vi "RelayBoard_16in16out_ZQ.vi"() -> ()   [LabVIEW 2013]
uses:
  <vilib>/Instr/_visa.llb/VISA Configure Serial Port (Instr).vi
panel:
  out "数组 2":bool[](array[boolean])
  out "数组":bool[](array[boolean])
  out "连接状态":bool
  in  "全部断开":bool
  in  "全部闭合":bool
  in  "OUT 16":bool
  in  "OUT 15":bool
  in  "OUT 14":bool
  in  "OUT 13":bool
  in  "OUT 12":bool
  in  "OUT 11":bool
  in  "OUT 10":bool
  in  "OUT 9":bool
  in  "OUT 8":bool
  in  "OUT 7":bool
  in  "OUT 6":bool
  in  "OUT 5":bool
  in  "OUT 4":bool
  in  "OUT 3":bool
  in  "打开端口":bool
  in  "停止":bool
  in  "OUT 2":bool
  in  "OUT 1":bool
  in  "VISA resource name":refnum<visa-resource-name> caption="VISA资源名称"
  # "X1"
  # "X2"
  # "X3"
  # "X4"
  # "X5"
  # "X6"
  # "X7"
  # "X8"
  # "X9"
  # "X10"
  # "X11"
  # "X12"
  # "X13"
  # "X14"
  # "X15"
  # "X16"
  # "X1"
  # "X2"
  # "X3"
  # "X4"
  # "X5"
  # "X6"
  # "X7"
  # "X8"
  # "X9"
  # "X10"
  # "X11"
  # "X12"
  # "X13"
  # "X14"
  # "X15"
  # "X16"
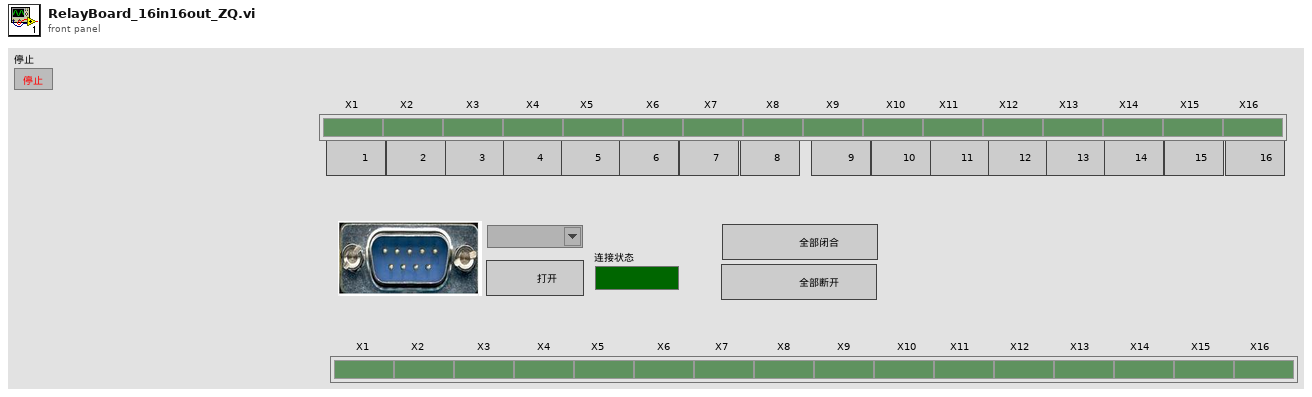
[diagram p1: front panel]
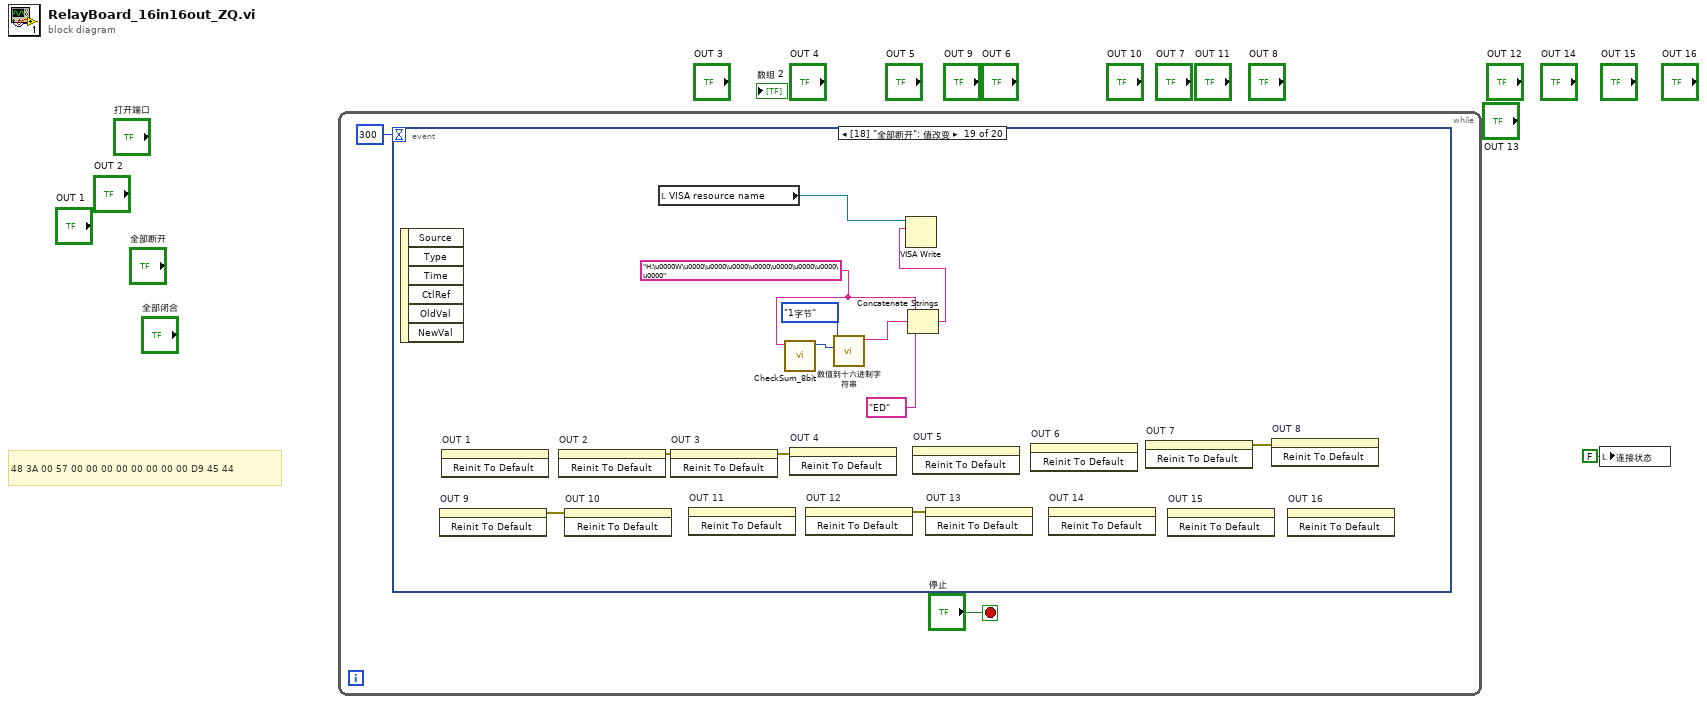
[diagram p0: block diagram]
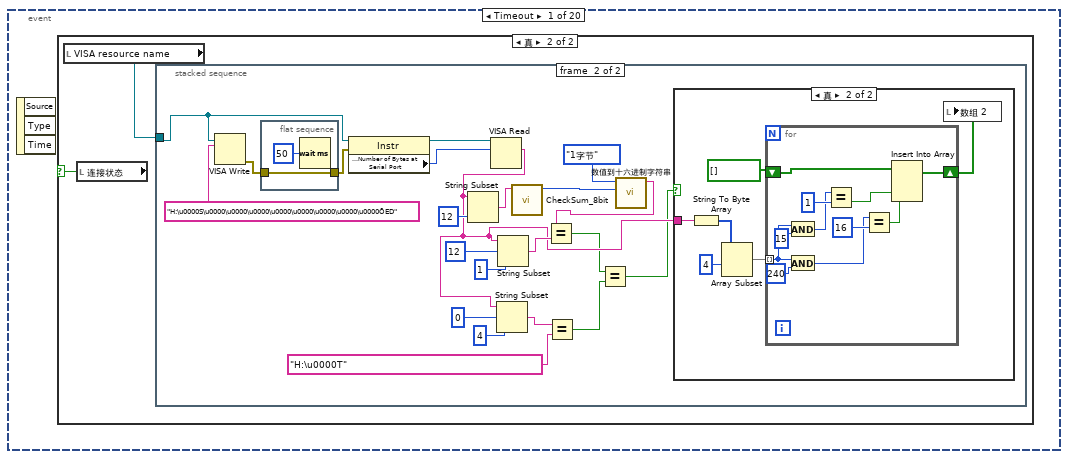
[diagram p2: hidden frame]
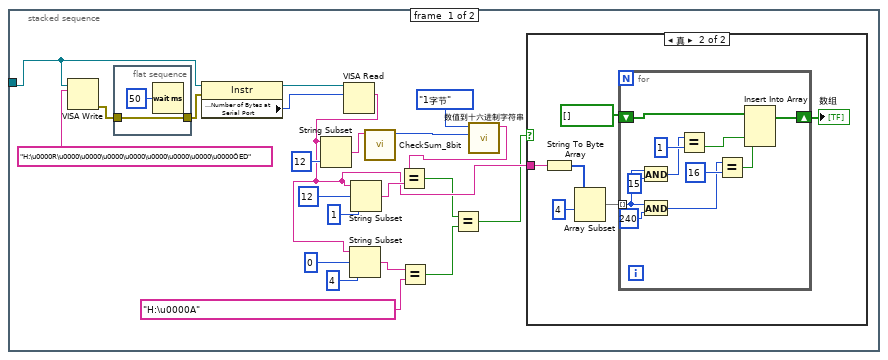
[diagram p4: hidden frame]
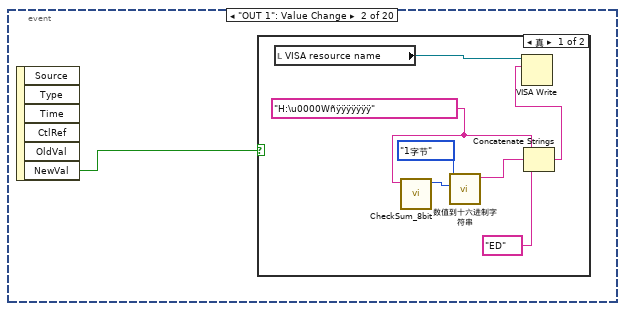
[diagram p7: hidden frame]
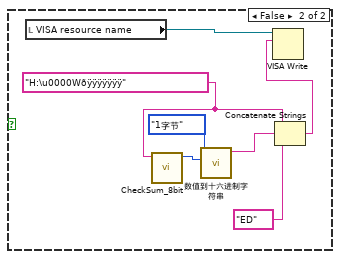
[diagram p8: hidden frame]
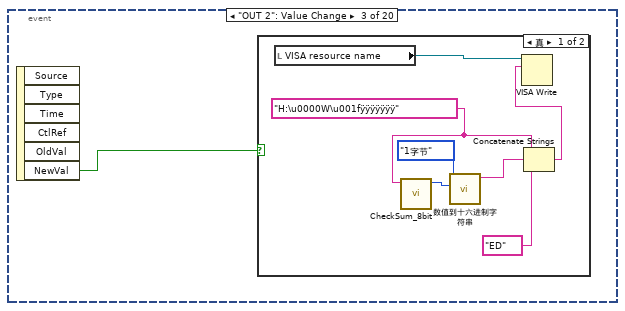
[diagram p9: hidden frame]
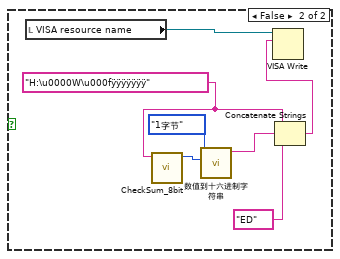
[diagram p10: hidden frame]
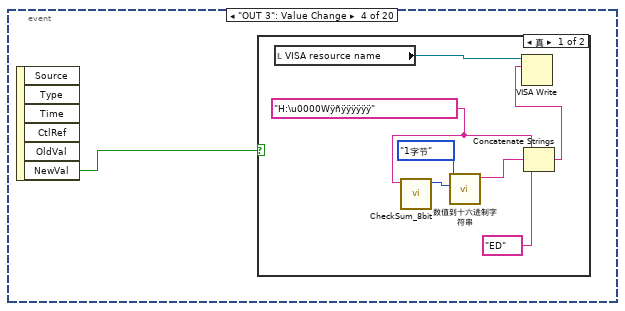
[diagram p11: hidden frame]
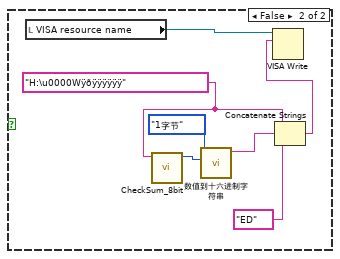
[diagram p12: hidden frame]
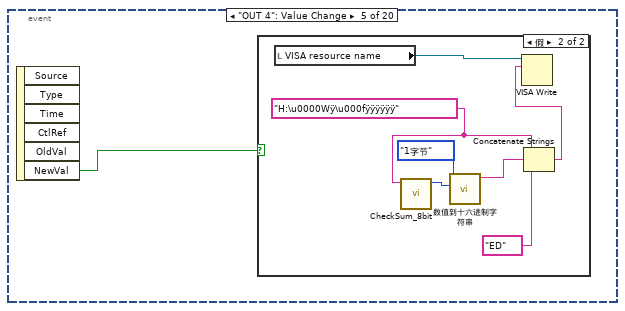
[diagram p13: hidden frame]
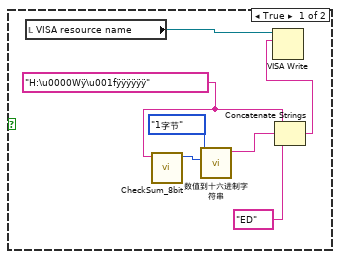
[diagram p14: hidden frame]
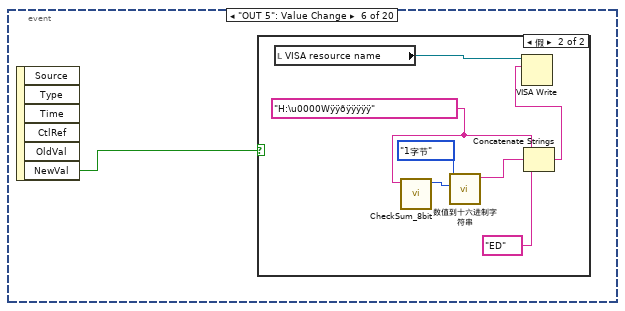
[diagram p15: hidden frame]
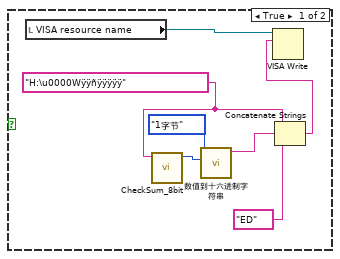
[diagram p16: hidden frame]
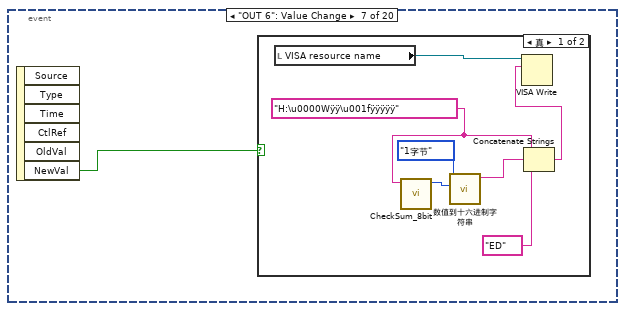
[diagram p17: hidden frame]
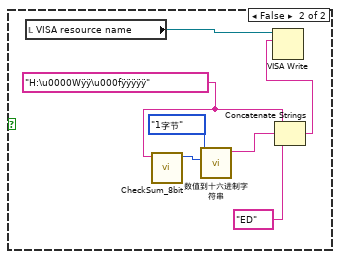
[diagram p18: hidden frame]
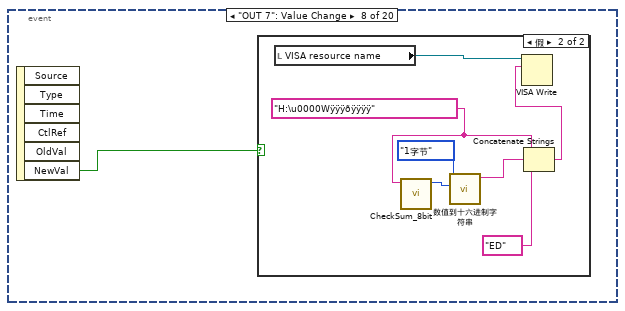
[diagram p19: hidden frame]
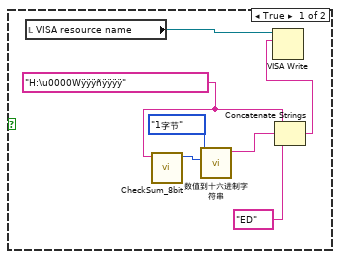
[diagram p20: hidden frame]
diagram:
  # "48 3A 00 57 00 00 00 00 00 00 00 00 D9 45 44"
  n1 = while {
    stop <- "停止" stop-if-true
    n2 = event shown="[18] \"全部断开\": 值改变" {
      selector: _ -> [_ _ _ _ _ _ _ _ _ _ _ _ _ _ _ _ _ _ _ _]
      dyn-events: _ -> [_ _ _ _ _ _ _ _ _ _ _ _ _ _ _ _ _ _ _ _]
      timeout: 300 -> [_ _ _ _ _ _ _ _ _ _ _ _ _ _ _ _ _ _ _ _]
      event Timeout {
        n3 = event-data() -> ()  [unwired: 1 in, 3 out]
        n4 = local read "连接状态"() -> (w4:bool)
        n5 = case shown="真" w4 {
          frame False {
          }
          frame True {
            n6 = local read "VISA resource name"() -> (w5:refnum<visa-resource-name>)
            n7 = stacked-sequence {
              tunnel: w5 -> [w22 w63]
              frame #0 {
                n8 = VISA Write(VISA resource name=w22, write buffer="H:\u0000R\u0000\u0000\u0000\u0000\u0000\u0000\u0000\u0000ÔED" ("写入缓冲区")) -> (error out=w23:errorcluster)  [unwired: 1 in, 2 out]
                n9 = flat-sequence {
                  tunnel: [w28] -> w24
                  tunnel: w23 -> [w28]
                  frame #0 {
                    n10 = Wait (ms)(milliseconds to wait=u32 50 ("等待时间（毫秒）")) -> ()  [unwired: 1 out]
                  }
                }
                n11 = property class="Instr"(reference=w22, error in=w24) -> (reference out=w27:refnum<visa-resource-name>, "Serial Settings:Number of Bytes at Serial Port"=w26:u32)  [unwired: 1 out]
                n12 = VISA Read(VISA resource name=w27, byte count=w26) -> (read buffer=w11:string)  [unwired: 1 in, 3 out]
                n13 = String Subset(string=w11, length (rest)=12 ("长度（剩余）")) -> (substring=w17:string)  [unwired: 1 in]
                n14 = String Subset(string=w11, offset (0)=0 ("偏移量(0)"), length (rest)=4 ("长度（剩余）")) -> (substring=w10:string)
                n15 = String Subset(string=w11, offset (0)=12 ("偏移量(0)"), length (rest)=1 ("长度（剩余）")) -> (substring=w18:string)
                n16 = call "CheckSum_8bit.vi"("字符串"=w17) -> ("和"=w15:u32)  [unwired: 10 in]
                n17 = Equal?(x=w10, y="H:\u0000A" ("写入缓冲区")) -> (x = y?=w7:bool)
                n18 = call "数值到十六进制字符串.vi"("Numeric"=w15, "转换字节数"=enum16{"1字节", "2字节", "4字节", "3字节"}."1字节") -> ("转换结果"=w14:string)  [unwired: 8 in, 1 out]
                n19 = Equal?(x=w14, y=w18) -> (x = y?=w8:bool)
                n20 = Equal?(x=w8, y=w7) -> (x = y?=w6:bool)
                n21 = case shown="真" w6 {
                  tunnel: w11 -> [_ w35]
                  frame False {
                  }
                  frame True {
                    n22 = String To Byte Array(string=w35) -> (unsigned byte array=w34:u8[])
                    n23 = Array Subset(array=w34, index=4 ("索引")) -> (w32:u8[])  [unwired: 1 in]
                    n24 = for {
                      tunnel: w32 -> [w39] mode=indexing
                      shift-right: [w41] -> w30
                      shift-left: bool[] [] -> [w44]
                      n25 = And(x=w39, y=u8 15) -> (x .and. y?=w37:u8)
                      n26 = And(x=w39, y=u8 240) -> (x .and. y?=w36:u8)
                      n27 = Equal?(x=w37, y=u8 1) -> (x = y?=w43:bool)
                      n28 = Equal?(x=w36, y=u8 16) -> (x = y?=w42:bool)
                      n29 = Insert Into Array(array=w44, new element #1=w43, new element #2=w42) -> (w41:bool[])  [unwired: 1 in]
                    }
                    "数组" <- w30
                  }
                }
              }
              frame #1 {
                n30 = VISA Write(VISA resource name=w63, write buffer="H:\u0000S\u0000\u0000\u0000\u0000\u0000\u0000\u0000\u0000ÕED" ("写入缓冲区")) -> (error out=w64:errorcluster)  [unwired: 1 in, 2 out]
                n31 = flat-sequence {
                  tunnel: [w69] -> w65
                  tunnel: w64 -> [w69]
                  frame #0 {
                    n32 = Wait (ms)(milliseconds to wait=u32 50 ("等待时间（毫秒）")) -> ()  [unwired: 1 out]
                  }
                }
                n33 = property class="Instr"(reference=w63, error in=w65) -> (reference out=w68:refnum<visa-resource-name>, "Serial Settings:Number of Bytes at Serial Port"=w67:u32)  [unwired: 1 out]
                n34 = VISA Read(VISA resource name=w68, byte count=w67) -> (read buffer=w52:string)  [unwired: 1 in, 3 out]
                n35 = String Subset(string=w52, length (rest)=12 ("长度（剩余）")) -> (substring=w58:string)  [unwired: 1 in]
                n36 = String Subset(string=w52, offset (0)=0 ("偏移量(0)"), length (rest)=4 ("长度（剩余）")) -> (substring=w51:string)
                n37 = String Subset(string=w52, offset (0)=12 ("偏移量(0)"), length (rest)=1 ("长度（剩余）")) -> (substring=w59:string)
                n38 = call "CheckSum_8bit.vi"("字符串"=w58) -> ("和"=w56:u32)  [unwired: 10 in]
                n39 = Equal?(x=w51, y="H:\u0000T" ("写入缓冲区")) -> (x = y?=w48:bool)
                n40 = call "数值到十六进制字符串.vi"("Numeric"=w56, "转换字节数"=enum16{"1字节", "2字节", "4字节", "3字节"}."1字节") -> ("转换结果"=w55:string)  [unwired: 8 in, 1 out]
                n41 = Equal?(x=w55, y=w59) -> (x = y?=w49:bool)
                n42 = Equal?(x=w49, y=w48) -> (x = y?=w47:bool)
                n43 = case shown="真" w47 {
                  tunnel: w52 -> [_ w76]
                  frame False {
                  }
                  frame True {
                    n44 = String To Byte Array(string=w76) -> (unsigned byte array=w75:u8[])
                    n45 = Array Subset(array=w75, index=4 ("索引")) -> (w73:u8[])  [unwired: 1 in]
                    n46 = for {
                      tunnel: w73 -> [w80] mode=indexing
                      shift-right: [w82] -> w71
                      shift-left: bool[] [] -> [w85]
                      n47 = And(x=w80, y=u8 15) -> (x .and. y?=w78:u8)
                      n48 = And(x=w80, y=u8 240) -> (x .and. y?=w77:u8)
                      n49 = Equal?(x=w78, y=u8 1) -> (x = y?=w84:bool)
                      n50 = Equal?(x=w77, y=u8 16) -> (x = y?=w83:bool)
                      n51 = Insert Into Array(array=w85, new element #1=w84, new element #2=w83) -> (w82:bool[])  [unwired: 1 in]
                    }
                    n52 = local write "数组 2"(w71) -> ()
                  }
                }
              }
            }
          }
        }
      }
      event "OUT 1": Value Change {
        n53 = event-data() -> ("NewVal"=w88:bool)  [unwired: 1 in, 5 out]
        n54 = case shown="真" w88 {
          frame True {
            w89 = "H:\u0000Wñÿÿÿÿÿÿÿ" ("写入缓冲区")
            n55 = local read "VISA resource name"() -> (w95:refnum<visa-resource-name>)
            n56 = call "CheckSum_8bit.vi"("字符串"=w89) -> ("和"=w94:u32)  [unwired: 10 in]
            n57 = call "数值到十六进制字符串.vi"("Numeric"=w94, "转换字节数"=enum16{"1字节", "2字节", "4字节", "3字节"}."1字节") -> ("转换结果"=w92:string)  [unwired: 8 in, 1 out]
            n58 = Concatenate Strings(w89, w92, "ED" ("写入缓冲区")) -> (w90:string)
            n59 = VISA Write(VISA resource name=w95, write buffer=w90) -> ()  [unwired: 1 in, 3 out]
          }
          frame False {
            w96 = "H:\u0000Wðÿÿÿÿÿÿÿ" ("写入缓冲区")
            n60 = local read "VISA resource name"() -> (w102:refnum<visa-resource-name>)
            n61 = call "CheckSum_8bit.vi"("字符串"=w96) -> ("和"=w101:u32)  [unwired: 10 in]
            n62 = call "数值到十六进制字符串.vi"("Numeric"=w101, "转换字节数"=enum16{"1字节", "2字节", "4字节", "3字节"}."1字节") -> ("转换结果"=w99:string)  [unwired: 8 in, 1 out]
            n63 = Concatenate Strings(w96, w99, "ED" ("写入缓冲区")) -> (w97:string)
            n64 = VISA Write(VISA resource name=w102, write buffer=w97) -> ()  [unwired: 1 in, 3 out]
          }
        }
      }
      event "OUT 2": Value Change {
        n65 = event-data() -> ("NewVal"=w103:bool)  [unwired: 1 in, 5 out]
        n66 = case shown="真" w103 {
          frame True {
            w104 = "H:\u0000W\u001fÿÿÿÿÿÿÿ" ("写入缓冲区")
            n67 = local read "VISA resource name"() -> (w110:refnum<visa-resource-name>)
            n68 = call "CheckSum_8bit.vi"("字符串"=w104) -> ("和"=w109:u32)  [unwired: 10 in]
            n69 = call "数值到十六进制字符串.vi"("Numeric"=w109, "转换字节数"=enum16{"1字节", "2字节", "4字节", "3字节"}."1字节") -> ("转换结果"=w107:string)  [unwired: 8 in, 1 out]
            n70 = Concatenate Strings(w104, w107, "ED" ("写入缓冲区")) -> (w105:string)
            n71 = VISA Write(VISA resource name=w110, write buffer=w105) -> ()  [unwired: 1 in, 3 out]
          }
          frame False {
            w111 = "H:\u0000W\u000fÿÿÿÿÿÿÿ" ("写入缓冲区")
            n72 = local read "VISA resource name"() -> (w117:refnum<visa-resource-name>)
            n73 = call "CheckSum_8bit.vi"("字符串"=w111) -> ("和"=w116:u32)  [unwired: 10 in]
            n74 = call "数值到十六进制字符串.vi"("Numeric"=w116, "转换字节数"=enum16{"1字节", "2字节", "4字节", "3字节"}."1字节") -> ("转换结果"=w114:string)  [unwired: 8 in, 1 out]
            n75 = Concatenate Strings(w111, w114, "ED" ("写入缓冲区")) -> (w112:string)
            n76 = VISA Write(VISA resource name=w117, write buffer=w112) -> ()  [unwired: 1 in, 3 out]
          }
        }
      }
      event "OUT 3": Value Change {
        n77 = event-data() -> ("NewVal"=w118:bool)  [unwired: 1 in, 5 out]
        n78 = case shown="真" w118 {
          frame True {
            w119 = "H:\u0000Wÿñÿÿÿÿÿÿ" ("写入缓冲区")
            n79 = local read "VISA resource name"() -> (w125:refnum<visa-resource-name>)
            n80 = call "CheckSum_8bit.vi"("字符串"=w119) -> ("和"=w124:u32)  [unwired: 10 in]
            n81 = call "数值到十六进制字符串.vi"("Numeric"=w124, "转换字节数"=enum16{"1字节", "2字节", "4字节", "3字节"}."1字节") -> ("转换结果"=w122:string)  [unwired: 8 in, 1 out]
            n82 = Concatenate Strings(w119, w122, "ED" ("写入缓冲区")) -> (w120:string)
            n83 = VISA Write(VISA resource name=w125, write buffer=w120) -> ()  [unwired: 1 in, 3 out]
          }
          frame False {
            w126 = "H:\u0000Wÿðÿÿÿÿÿÿ" ("写入缓冲区")
            n84 = local read "VISA resource name"() -> (w132:refnum<visa-resource-name>)
            n85 = call "CheckSum_8bit.vi"("字符串"=w126) -> ("和"=w131:u32)  [unwired: 10 in]
            n86 = call "数值到十六进制字符串.vi"("Numeric"=w131, "转换字节数"=enum16{"1字节", "2字节", "4字节", "3字节"}."1字节") -> ("转换结果"=w129:string)  [unwired: 8 in, 1 out]
            n87 = Concatenate Strings(w126, w129, "ED" ("写入缓冲区")) -> (w127:string)
            n88 = VISA Write(VISA resource name=w132, write buffer=w127) -> ()  [unwired: 1 in, 3 out]
          }
        }
      }
      event "OUT 4": Value Change {
        n89 = event-data() -> ("NewVal"=w133:bool)  [unwired: 1 in, 5 out]
        n90 = case shown="假" w133 {
          frame True {
            w134 = "H:\u0000Wÿ\u001fÿÿÿÿÿÿ" ("写入缓冲区")
            n91 = local read "VISA resource name"() -> (w140:refnum<visa-resource-name>)
            n92 = call "CheckSum_8bit.vi"("字符串"=w134) -> ("和"=w139:u32)  [unwired: 10 in]
            n93 = call "数值到十六进制字符串.vi"("Numeric"=w139, "转换字节数"=enum16{"1字节", "2字节", "4字节", "3字节"}."1字节") -> ("转换结果"=w137:string)  [unwired: 8 in, 1 out]
            n94 = Concatenate Strings(w134, w137, "ED" ("写入缓冲区")) -> (w135:string)
            n95 = VISA Write(VISA resource name=w140, write buffer=w135) -> ()  [unwired: 1 in, 3 out]
          }
          frame False {
            w141 = "H:\u0000Wÿ\u000fÿÿÿÿÿÿ" ("写入缓冲区")
            n96 = local read "VISA resource name"() -> (w147:refnum<visa-resource-name>)
            n97 = call "CheckSum_8bit.vi"("字符串"=w141) -> ("和"=w146:u32)  [unwired: 10 in]
            n98 = call "数值到十六进制字符串.vi"("Numeric"=w146, "转换字节数"=enum16{"1字节", "2字节", "4字节", "3字节"}."1字节") -> ("转换结果"=w144:string)  [unwired: 8 in, 1 out]
            n99 = Concatenate Strings(w141, w144, "ED" ("写入缓冲区")) -> (w142:string)
            n100 = VISA Write(VISA resource name=w147, write buffer=w142) -> ()  [unwired: 1 in, 3 out]
          }
        }
      }
      event "OUT 5": Value Change {
        n101 = event-data() -> ("NewVal"=w148:bool)  [unwired: 1 in, 5 out]
        n102 = case shown="假" w148 {
          frame True {
            w149 = "H:\u0000Wÿÿñÿÿÿÿÿ" ("写入缓冲区")
            n103 = local read "VISA resource name"() -> (w155:refnum<visa-resource-name>)
            n104 = call "CheckSum_8bit.vi"("字符串"=w149) -> ("和"=w154:u32)  [unwired: 10 in]
            n105 = call "数值到十六进制字符串.vi"("Numeric"=w154, "转换字节数"=enum16{"1字节", "2字节", "4字节", "3字节"}."1字节") -> ("转换结果"=w152:string)  [unwired: 8 in, 1 out]
            n106 = Concatenate Strings(w149, w152, "ED" ("写入缓冲区")) -> (w150:string)
            n107 = VISA Write(VISA resource name=w155, write buffer=w150) -> ()  [unwired: 1 in, 3 out]
          }
          frame False {
            w156 = "H:\u0000Wÿÿðÿÿÿÿÿ" ("写入缓冲区")
            n108 = local read "VISA resource name"() -> (w162:refnum<visa-resource-name>)
            n109 = call "CheckSum_8bit.vi"("字符串"=w156) -> ("和"=w161:u32)  [unwired: 10 in]
            n110 = call "数值到十六进制字符串.vi"("Numeric"=w161, "转换字节数"=enum16{"1字节", "2字节", "4字节", "3字节"}."1字节") -> ("转换结果"=w159:string)  [unwired: 8 in, 1 out]
            n111 = Concatenate Strings(w156, w159, "ED" ("写入缓冲区")) -> (w157:string)
            n112 = VISA Write(VISA resource name=w162, write buffer=w157) -> ()  [unwired: 1 in, 3 out]
          }
        }
      }
      event "OUT 6": Value Change {
        n113 = event-data() -> ("NewVal"=w163:bool)  [unwired: 1 in, 5 out]
        n114 = case shown="真" w163 {
          frame True {
            w164 = "H:\u0000Wÿÿ\u001fÿÿÿÿÿ" ("写入缓冲区")
            n115 = local read "VISA resource name"() -> (w170:refnum<visa-resource-name>)
            n116 = call "CheckSum_8bit.vi"("字符串"=w164) -> ("和"=w169:u32)  [unwired: 10 in]
            n117 = call "数值到十六进制字符串.vi"("Numeric"=w169, "转换字节数"=enum16{"1字节", "2字节", "4字节", "3字节"}."1字节") -> ("转换结果"=w167:string)  [unwired: 8 in, 1 out]
            n118 = Concatenate Strings(w164, w167, "ED" ("写入缓冲区")) -> (w165:string)
            n119 = VISA Write(VISA resource name=w170, write buffer=w165) -> ()  [unwired: 1 in, 3 out]
          }
          frame False {
            w171 = "H:\u0000Wÿÿ\u000fÿÿÿÿÿ" ("写入缓冲区")
            n120 = local read "VISA resource name"() -> (w177:refnum<visa-resource-name>)
            n121 = call "CheckSum_8bit.vi"("字符串"=w171) -> ("和"=w176:u32)  [unwired: 10 in]
            n122 = call "数值到十六进制字符串.vi"("Numeric"=w176, "转换字节数"=enum16{"1字节", "2字节", "4字节", "3字节"}."1字节") -> ("转换结果"=w174:string)  [unwired: 8 in, 1 out]
            n123 = Concatenate Strings(w171, w174, "ED" ("写入缓冲区")) -> (w172:string)
            n124 = VISA Write(VISA resource name=w177, write buffer=w172) -> ()  [unwired: 1 in, 3 out]
          }
        }
      }
      event "OUT 7": Value Change {
        n125 = event-data() -> ("NewVal"=w178:bool)  [unwired: 1 in, 5 out]
        n126 = case shown="假" w178 {
          frame True {
            w179 = "H:\u0000Wÿÿÿñÿÿÿÿ" ("写入缓冲区")
            n127 = local read "VISA resource name"() -> (w185:refnum<visa-resource-name>)
            n128 = call "CheckSum_8bit.vi"("字符串"=w179) -> ("和"=w184:u32)  [unwired: 10 in]
            n129 = call "数值到十六进制字符串.vi"("Numeric"=w184, "转换字节数"=enum16{"1字节", "2字节", "4字节", "3字节"}."1字节") -> ("转换结果"=w182:string)  [unwired: 8 in, 1 out]
            n130 = Concatenate Strings(w179, w182, "ED" ("写入缓冲区")) -> (w180:string)
            n131 = VISA Write(VISA resource name=w185, write buffer=w180) -> ()  [unwired: 1 in, 3 out]
          }
          frame False {
            w186 = "H:\u0000Wÿÿÿðÿÿÿÿ" ("写入缓冲区")
            n132 = local read "VISA resource name"() -> (w192:refnum<visa-resource-name>)
            n133 = call "CheckSum_8bit.vi"("字符串"=w186) -> ("和"=w191:u32)  [unwired: 10 in]
            n134 = call "数值到十六进制字符串.vi"("Numeric"=w191, "转换字节数"=enum16{"1字节", "2字节", "4字节", "3字节"}."1字节") -> ("转换结果"=w189:string)  [unwired: 8 in, 1 out]
            n135 = Concatenate Strings(w186, w189, "ED" ("写入缓冲区")) -> (w187:string)
            n136 = VISA Write(VISA resource name=w192, write buffer=w187) -> ()  [unwired: 1 in, 3 out]
          }
        }
      }
      event "OUT 8": Value Change {
        n137 = event-data() -> ("NewVal"=w193:bool)  [unwired: 1 in, 5 out]
        n138 = case shown="真" w193 {
          frame True {
            w194 = "H:\u0000Wÿÿÿ\u001fÿÿÿÿ" ("写入缓冲区")
            n139 = local read "VISA resource name"() -> (w200:refnum<visa-resource-name>)
            n140 = call "CheckSum_8bit.vi"("字符串"=w194) -> ("和"=w199:u32)  [unwired: 10 in]
            n141 = call "数值到十六进制字符串.vi"("Numeric"=w199, "转换字节数"=enum16{"1字节", "2字节", "4字节", "3字节"}."1字节") -> ("转换结果"=w197:string)  [unwired: 8 in, 1 out]
            n142 = Concatenate Strings(w194, w197, "ED" ("写入缓冲区")) -> (w195:string)
            n143 = VISA Write(VISA resource name=w200, write buffer=w195) -> ()  [unwired: 1 in, 3 out]
          }
          frame False {
            w201 = "H:\u0000Wÿÿÿ\u000fÿÿÿÿ" ("写入缓冲区")
            n144 = local read "VISA resource name"() -> (w207:refnum<visa-resource-name>)
            n145 = call "CheckSum_8bit.vi"("字符串"=w201) -> ("和"=w206:u32)  [unwired: 10 in]
            n146 = call "数值到十六进制字符串.vi"("Numeric"=w206, "转换字节数"=enum16{"1字节", "2字节", "4字节", "3字节"}."1字节") -> ("转换结果"=w204:string)  [unwired: 8 in, 1 out]
            n147 = Concatenate Strings(w201, w204, "ED" ("写入缓冲区")) -> (w202:string)
            n148 = VISA Write(VISA resource name=w207, write buffer=w202) -> ()  [unwired: 1 in, 3 out]
          }
        }
      }
      event "OUT 9": Value Change {
        n149 = event-data() -> ("NewVal"=w208:bool)  [unwired: 1 in, 5 out]
        n150 = case shown="真" w208 {
          frame True {
            w209 = "H:\u0000Wÿÿÿÿñÿÿÿ" ("写入缓冲区")
            n151 = local read "VISA resource name"() -> (w215:refnum<visa-resource-name>)
            n152 = call "CheckSum_8bit.vi"("字符串"=w209) -> ("和"=w214:u32)  [unwired: 10 in]
            n153 = call "数值到十六进制字符串.vi"("Numeric"=w214, "转换字节数"=enum16{"1字节", "2字节", "4字节", "3字节"}."1字节") -> ("转换结果"=w212:string)  [unwired: 8 in, 1 out]
            n154 = Concatenate Strings(w209, w212, "ED" ("写入缓冲区")) -> (w210:string)
            n155 = VISA Write(VISA resource name=w215, write buffer=w210) -> ()  [unwired: 1 in, 3 out]
          }
          frame False {
            w216 = "H:\u0000Wÿÿÿÿðÿÿÿ" ("写入缓冲区")
            n156 = local read "VISA resource name"() -> (w222:refnum<visa-resource-name>)
            n157 = call "CheckSum_8bit.vi"("字符串"=w216) -> ("和"=w221:u32)  [unwired: 10 in]
            n158 = call "数值到十六进制字符串.vi"("Numeric"=w221, "转换字节数"=enum16{"1字节", "2字节", "4字节", "3字节"}."1字节") -> ("转换结果"=w219:string)  [unwired: 8 in, 1 out]
            n159 = Concatenate Strings(w216, w219, "ED" ("写入缓冲区")) -> (w217:string)
            n160 = VISA Write(VISA resource name=w222, write buffer=w217) -> ()  [unwired: 1 in, 3 out]
          }
        }
      }
      event "OUT 10": Value Change {
        n161 = event-data() -> ("NewVal"=w223:bool)  [unwired: 1 in, 5 out]
        n162 = case shown="假" w223 {
          frame True {
            w224 = "H:\u0000Wÿÿÿÿ\u001fÿÿÿ" ("写入缓冲区")
            n163 = local read "VISA resource name"() -> (w230:refnum<visa-resource-name>)
            n164 = call "CheckSum_8bit.vi"("字符串"=w224) -> ("和"=w229:u32)  [unwired: 10 in]
            n165 = call "数值到十六进制字符串.vi"("Numeric"=w229, "转换字节数"=enum16{"1字节", "2字节", "4字节", "3字节"}."1字节") -> ("转换结果"=w227:string)  [unwired: 8 in, 1 out]
            n166 = Concatenate Strings(w224, w227, "ED" ("写入缓冲区")) -> (w225:string)
            n167 = VISA Write(VISA resource name=w230, write buffer=w225) -> ()  [unwired: 1 in, 3 out]
          }
          frame False {
            w231 = "H:\u0000Wÿÿÿÿ\u000fÿÿÿ" ("写入缓冲区")
            n168 = local read "VISA resource name"() -> (w237:refnum<visa-resource-name>)
            n169 = call "CheckSum_8bit.vi"("字符串"=w231) -> ("和"=w236:u32)  [unwired: 10 in]
            n170 = call "数值到十六进制字符串.vi"("Numeric"=w236, "转换字节数"=enum16{"1字节", "2字节", "4字节", "3字节"}."1字节") -> ("转换结果"=w234:string)  [unwired: 8 in, 1 out]
            n171 = Concatenate Strings(w231, w234, "ED" ("写入缓冲区")) -> (w232:string)
            n172 = VISA Write(VISA resource name=w237, write buffer=w232) -> ()  [unwired: 1 in, 3 out]
          }
        }
      }
      event "OUT 11": Value Change {
        n173 = event-data() -> ("NewVal"=w238:bool)  [unwired: 1 in, 5 out]
        n174 = case shown="假" w238 {
          frame True {
            w239 = "H:\u0000Wÿÿÿÿÿñÿÿ" ("写入缓冲区")
            n175 = local read "VISA resource name"() -> (w245:refnum<visa-resource-name>)
            n176 = call "CheckSum_8bit.vi"("字符串"=w239) -> ("和"=w244:u32)  [unwired: 10 in]
            n177 = call "数值到十六进制字符串.vi"("Numeric"=w244, "转换字节数"=enum16{"1字节", "2字节", "4字节", "3字节"}."1字节") -> ("转换结果"=w242:string)  [unwired: 8 in, 1 out]
            n178 = Concatenate Strings(w239, w242, "ED" ("写入缓冲区")) -> (w240:string)
            n179 = VISA Write(VISA resource name=w245, write buffer=w240) -> ()  [unwired: 1 in, 3 out]
          }
          frame False {
            w246 = "H:\u0000Wÿÿÿÿÿðÿÿ" ("写入缓冲区")
            n180 = local read "VISA resource name"() -> (w252:refnum<visa-resource-name>)
            n181 = call "CheckSum_8bit.vi"("字符串"=w246) -> ("和"=w251:u32)  [unwired: 10 in]
            n182 = call "数值到十六进制字符串.vi"("Numeric"=w251, "转换字节数"=enum16{"1字节", "2字节", "4字节", "3字节"}."1字节") -> ("转换结果"=w249:string)  [unwired: 8 in, 1 out]
            n183 = Concatenate Strings(w246, w249, "ED" ("写入缓冲区")) -> (w247:string)
            n184 = VISA Write(VISA resource name=w252, write buffer=w247) -> ()  [unwired: 1 in, 3 out]
          }
        }
      }
      event "OUT 12": Value Change {
        n185 = event-data() -> ("NewVal"=w253:bool)  [unwired: 1 in, 5 out]
        n186 = case shown="真" w253 {
          frame True {
            w254 = "H:\u0000Wÿÿÿÿÿ\u001fÿÿ" ("写入缓冲区")
            n187 = local read "VISA resource name"() -> (w260:refnum<visa-resource-name>)
            n188 = call "CheckSum_8bit.vi"("字符串"=w254) -> ("和"=w259:u32)  [unwired: 10 in]
            n189 = call "数值到十六进制字符串.vi"("Numeric"=w259, "转换字节数"=enum16{"1字节", "2字节", "4字节", "3字节"}."1字节") -> ("转换结果"=w257:string)  [unwired: 8 in, 1 out]
            n190 = Concatenate Strings(w254, w257, "ED" ("写入缓冲区")) -> (w255:string)
            n191 = VISA Write(VISA resource name=w260, write buffer=w255) -> ()  [unwired: 1 in, 3 out]
          }
          frame False {
            w261 = "H:\u0000Wÿÿÿÿÿ\u000fÿÿ" ("写入缓冲区")
            n192 = local read "VISA resource name"() -> (w267:refnum<visa-resource-name>)
            n193 = call "CheckSum_8bit.vi"("字符串"=w261) -> ("和"=w266:u32)  [unwired: 10 in]
            n194 = call "数值到十六进制字符串.vi"("Numeric"=w266, "转换字节数"=enum16{"1字节", "2字节", "4字节", "3字节"}."1字节") -> ("转换结果"=w264:string)  [unwired: 8 in, 1 out]
            n195 = Concatenate Strings(w261, w264, "ED" ("写入缓冲区")) -> (w262:string)
            n196 = VISA Write(VISA resource name=w267, write buffer=w262) -> ()  [unwired: 1 in, 3 out]
          }
        }
      }
      event "OUT 13": Value Change {
        n197 = event-data() -> ("NewVal"=w268:bool)  [unwired: 1 in, 5 out]
        n198 = case shown="真" w268 {
          frame True {
            w269 = "H:\u0000Wÿÿÿÿÿÿñÿ" ("写入缓冲区")
            n199 = local read "VISA resource name"() -> (w275:refnum<visa-resource-name>)
            n200 = call "CheckSum_8bit.vi"("字符串"=w269) -> ("和"=w274:u32)  [unwired: 10 in]
            n201 = call "数值到十六进制字符串.vi"("Numeric"=w274, "转换字节数"=enum16{"1字节", "2字节", "4字节", "3字节"}."1字节") -> ("转换结果"=w272:string)  [unwired: 8 in, 1 out]
            n202 = Concatenate Strings(w269, w272, "ED" ("写入缓冲区")) -> (w270:string)
            n203 = VISA Write(VISA resource name=w275, write buffer=w270) -> ()  [unwired: 1 in, 3 out]
          }
          frame False {
            w276 = "H:\u0000Wÿÿÿÿÿÿðÿ" ("写入缓冲区")
            n204 = local read "VISA resource name"() -> (w282:refnum<visa-resource-name>)
            n205 = call "CheckSum_8bit.vi"("字符串"=w276) -> ("和"=w281:u32)  [unwired: 10 in]
            n206 = call "数值到十六进制字符串.vi"("Numeric"=w281, "转换字节数"=enum16{"1字节", "2字节", "4字节", "3字节"}."1字节") -> ("转换结果"=w279:string)  [unwired: 8 in, 1 out]
            n207 = Concatenate Strings(w276, w279, "ED" ("写入缓冲区")) -> (w277:string)
            n208 = VISA Write(VISA resource name=w282, write buffer=w277) -> ()  [unwired: 1 in, 3 out]
          }
        }
      }
      event "OUT 14": Value Change {
        n209 = event-data() -> ("NewVal"=w283:bool)  [unwired: 1 in, 5 out]
        n210 = case shown="假" w283 {
          frame True {
            w284 = "H:\u0000Wÿÿÿÿÿÿ\u001fÿ" ("写入缓冲区")
            n211 = local read "VISA resource name"() -> (w290:refnum<visa-resource-name>)
            n212 = call "CheckSum_8bit.vi"("字符串"=w284) -> ("和"=w289:u32)  [unwired: 10 in]
            n213 = call "数值到十六进制字符串.vi"("Numeric"=w289, "转换字节数"=enum16{"1字节", "2字节", "4字节", "3字节"}."1字节") -> ("转换结果"=w287:string)  [unwired: 8 in, 1 out]
            n214 = Concatenate Strings(w284, w287, "ED" ("写入缓冲区")) -> (w285:string)
            n215 = VISA Write(VISA resource name=w290, write buffer=w285) -> ()  [unwired: 1 in, 3 out]
          }
          frame False {
            w291 = "H:\u0000Wÿÿÿÿÿÿ\u000fÿ" ("写入缓冲区")
            n216 = local read "VISA resource name"() -> (w297:refnum<visa-resource-name>)
            n217 = call "CheckSum_8bit.vi"("字符串"=w291) -> ("和"=w296:u32)  [unwired: 10 in]
            n218 = call "数值到十六进制字符串.vi"("Numeric"=w296, "转换字节数"=enum16{"1字节", "2字节", "4字节", "3字节"}."1字节") -> ("转换结果"=w294:string)  [unwired: 8 in, 1 out]
            n219 = Concatenate Strings(w291, w294, "ED" ("写入缓冲区")) -> (w292:string)
            n220 = VISA Write(VISA resource name=w297, write buffer=w292) -> ()  [unwired: 1 in, 3 out]
          }
        }
      }
      event "OUT 15": Value Change {
        n221 = event-data() -> ("NewVal"=w298:bool)  [unwired: 1 in, 5 out]
        n222 = case shown="真" w298 {
          frame True {
            w299 = "H:\u0000Wÿÿÿÿÿÿÿñ" ("写入缓冲区")
            n223 = local read "VISA resource name"() -> (w305:refnum<visa-resource-name>)
            n224 = call "CheckSum_8bit.vi"("字符串"=w299) -> ("和"=w304:u32)  [unwired: 10 in]
            n225 = call "数值到十六进制字符串.vi"("Numeric"=w304, "转换字节数"=enum16{"1字节", "2字节", "4字节", "3字节"}."1字节") -> ("转换结果"=w302:string)  [unwired: 8 in, 1 out]
            n226 = Concatenate Strings(w299, w302, "ED" ("写入缓冲区")) -> (w300:string)
            n227 = VISA Write(VISA resource name=w305, write buffer=w300) -> ()  [unwired: 1 in, 3 out]
          }
          frame False {
            w306 = "H:\u0000Wÿÿÿÿÿÿÿð" ("写入缓冲区")
            n228 = local read "VISA resource name"() -> (w312:refnum<visa-resource-name>)
            n229 = call "CheckSum_8bit.vi"("字符串"=w306) -> ("和"=w311:u32)  [unwired: 10 in]
            n230 = call "数值到十六进制字符串.vi"("Numeric"=w311, "转换字节数"=enum16{"1字节", "2字节", "4字节", "3字节"}."1字节") -> ("转换结果"=w309:string)  [unwired: 8 in, 1 out]
            n231 = Concatenate Strings(w306, w309, "ED" ("写入缓冲区")) -> (w307:string)
            n232 = VISA Write(VISA resource name=w312, write buffer=w307) -> ()  [unwired: 1 in, 3 out]
          }
        }
      }
      event "OUT 16": Value Change {
        n233 = event-data() -> ("NewVal"=w313:bool)  [unwired: 1 in, 5 out]
        n234 = case shown="假" w313 {
          frame True {
            w314 = "H:\u0000Wÿÿÿÿÿÿÿ\u001f" ("写入缓冲区")
            n235 = local read "VISA resource name"() -> (w320:refnum<visa-resource-name>)
            n236 = call "CheckSum_8bit.vi"("字符串"=w314) -> ("和"=w319:u32)  [unwired: 10 in]
            n237 = call "数值到十六进制字符串.vi"("Numeric"=w319, "转换字节数"=enum16{"1字节", "2字节", "4字节", "3字节"}."1字节") -> ("转换结果"=w317:string)  [unwired: 8 in, 1 out]
            n238 = Concatenate Strings(w314, w317, "ED" ("写入缓冲区")) -> (w315:string)
            n239 = VISA Write(VISA resource name=w320, write buffer=w315) -> ()  [unwired: 1 in, 3 out]
          }
          frame False {
            w321 = "H:\u0000Wÿÿÿÿÿÿÿ\u000f" ("写入缓冲区")
            n240 = local read "VISA resource name"() -> (w327:refnum<visa-resource-name>)
            n241 = call "CheckSum_8bit.vi"("字符串"=w321) -> ("和"=w326:u32)  [unwired: 10 in]
            n242 = call "数值到十六进制字符串.vi"("Numeric"=w326, "转换字节数"=enum16{"1字节", "2字节", "4字节", "3字节"}."1字节") -> ("转换结果"=w324:string)  [unwired: 8 in, 1 out]
            n243 = Concatenate Strings(w321, w324, "ED" ("写入缓冲区")) -> (w322:string)
            n244 = VISA Write(VISA resource name=w327, write buffer=w322) -> ()  [unwired: 1 in, 3 out]
          }
        }
      }
      event "全部闭合": Value Change {
        w328 = "H:\u0000W\u0011\u0011\u0011\u0011\u0011\u0011\u0011\u0011" ("写入缓冲区")
        n245 = event-data() -> ()  [unwired: 1 in, 6 out]
        n246 = local read "VISA resource name"() -> (w334:refnum<visa-resource-name>)
        n247 = call "CheckSum_8bit.vi"("字符串"=w328) -> ("和"=w333:u32)  [unwired: 10 in]
        n248 = call "数值到十六进制字符串.vi"("Numeric"=w333, "转换字节数"=enum16{"1字节", "2字节", "4字节", "3字节"}."1字节") -> ("转换结果"=w331:string)  [unwired: 8 in, 1 out]
        n249 = Concatenate Strings(w328, w331, "ED" ("写入缓冲区")) -> (w329:string)
        n250 = VISA Write(VISA resource name=w334, write buffer=w329) -> ()  [unwired: 1 in, 3 out]
      }
      event "全部断开": Value Change {
        w340 = "H:\u0000W\u0000\u0000\u0000\u0000\u0000\u0000\u0000\u0000" ("写入缓冲区")
        n251 = event-data() -> ()  [unwired: 1 in, 6 out]
        n252 = invoke on="OUT 9" class="Bool" method="Reinit To Default"() -> (error out=w336:errorcluster)  [unwired: 3 in, 2 out]
        n253 = invoke on="OUT 1" class="Bool" method="Reinit To Default"() -> ()  [unwired: 3 in, 3 out]
        n254 = invoke on="OUT 2" class="Bool" method="Reinit To Default"() -> (error out=w339:errorcluster)  [unwired: 3 in, 2 out]
        n255 = invoke on="OUT 10" class="Bool" method="Reinit To Default"(error in=w336) -> ()  [unwired: 2 in, 3 out]
        n256 = local read "VISA resource name"() -> (w346:refnum<visa-resource-name>)
        n257 = invoke on="OUT 3" class="Bool" method="Reinit To Default"(error in=w339) -> (error out=w338:errorcluster)  [unwired: 2 in, 2 out]
        n258 = invoke on="OUT 11" class="Bool" method="Reinit To Default"() -> ()  [unwired: 3 in, 3 out]
        n259 = call "CheckSum_8bit.vi"("字符串"=w340) -> ("和"=w345:u32)  [unwired: 10 in]
        n260 = invoke on="OUT 4" class="Bool" method="Reinit To Default"(error in=w338) -> ()  [unwired: 2 in, 3 out]
        n261 = invoke on="OUT 12" class="Bool" method="Reinit To Default"() -> (error out=w335:errorcluster)  [unwired: 3 in, 2 out]
        n262 = call "数值到十六进制字符串.vi"("Numeric"=w345, "转换字节数"=enum16{"1字节", "2字节", "4字节", "3字节"}."1字节") -> ("转换结果"=w343:string)  [unwired: 8 in, 1 out]
        n263 = Concatenate Strings(w340, w343, "ED" ("写入缓冲区")) -> (w341:string)
        n264 = VISA Write(VISA resource name=w346, write buffer=w341) -> ()  [unwired: 1 in, 3 out]
        n265 = invoke on="OUT 5" class="Bool" method="Reinit To Default"() -> ()  [unwired: 3 in, 3 out]
        n266 = invoke on="OUT 13" class="Bool" method="Reinit To Default"(error in=w335) -> ()  [unwired: 2 in, 3 out]
        n267 = invoke on="OUT 6" class="Bool" method="Reinit To Default"() -> ()  [unwired: 3 in, 3 out]
        n268 = invoke on="OUT 14" class="Bool" method="Reinit To Default"() -> ()  [unwired: 3 in, 3 out]
        n269 = invoke on="OUT 7" class="Bool" method="Reinit To Default"() -> (error out=w337:errorcluster)  [unwired: 3 in, 2 out]
        n270 = invoke on="OUT 15" class="Bool" method="Reinit To Default"() -> ()  [unwired: 3 in, 3 out]
        n271 = invoke on="OUT 8" class="Bool" method="Reinit To Default"(error in=w337) -> ()  [unwired: 2 in, 3 out]
        n272 = invoke on="OUT 16" class="Bool" method="Reinit To Default"() -> ()  [unwired: 3 in, 3 out]
      }
      event "打开端口": Value Change {
        n273 = event-data() -> ("NewVal"=w349:bool)  [unwired: 1 in, 5 out]
        n274 = case shown="假" w349 {
          tunnel: "VISA resource name" -> [w351 w356]
          tunnel: [w350 FALSE] -> w347
          frame True {
            n275 = call-poly "VISA Configure Serial Port"("VISA resource name"=w351, "baud rate (9600)"=u32 115200) -> ("error out"=w353:errorcluster)  [unwired: 12 in, 1 out]
            n276 = Unbundle(w353) -> ("status"=w352:bool)  [unwired: 2 out]
            n277 = Not(x=w352) -> (.not. x?=w350:bool)
          }
          frame False {
            n278 = VISA Close(VISA resource name=w356) -> ()  [unwired: 1 in, 1 out]
          }
        }
        "连接状态" <- w347
      }
    }
  }
  n279 = local write "连接状态"(FALSE ("status")) -> ()
